vi "filter signal.vi"(8 "error in (no error)":errorcluster, 11 "LineCCD in":refnum<class "LineCCD.lvclass">) -> (0 "error out":errorcluster, 3 "LineCCD out":refnum<class "LineCCD.lvclass">)   [LabVIEW 2012, in "LineCCD.lvclass"]
uses:
  LineCCD.lvclass
  LineCCD.lvclass/LineCCD.ctl
  <vilib>/Analysis/3filter.llb/Butterworth Filter (DBL).vi
  <vilib>/Analysis/NI_AALBase.lvlib
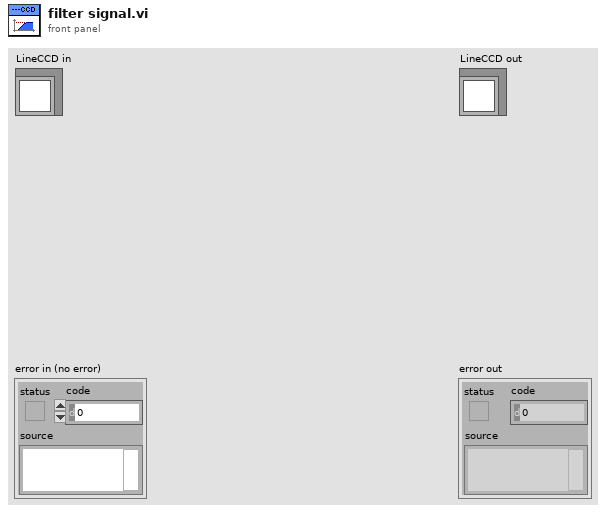
[diagram p1: front panel]
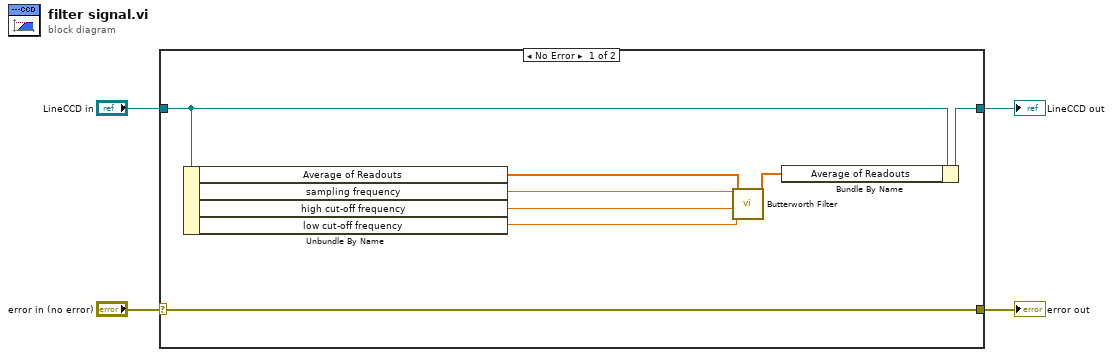
[diagram p0: block diagram]
diagram:
  n1 = case shown="No Error" "error in (no error)" {
    selector: "error in (no error)" -> [w12 w14]
    tunnel: [w12 w14] -> w3
    tunnel: [w10 w13] -> w1
    tunnel: "LineCCD in" -> [w11 w13]
    frame No Error {
      n2 = Unbundle By Name(w11) -> ("Average of Readouts"=w6:dbl[], "sampling frequency"=w9:dbl, "high cut-off frequency"=w8:dbl, "low cut-off frequency"=w7:dbl)
      n3 = call-poly <vilib>:"Butterworth Filter.vi"("low cutoff freq: fl"=w7, "high cutoff freq: fh"=w8, "sampling freq: fs"=w9, "X"=w6) -> ("Filtered X"=w5:dbl[])  [unwired: 4 in, 1 out]
      n4 = Bundle By Name(cluster=w11, "Average of Readouts"=w5) -> (w10:refnum<class "LineCCD.lvclass">)
    }
    frame Error {
    }
  }
  "error out" <- w3
  "LineCCD out" <- w1
